vi "NsimuladotTemp.vi"(9 "Lmin":dbl, 10 "Lmax":dbl, 11 "N":i32) -> (3 "Array":dbl[](array[numeric]))   [LabVIEW 2020]
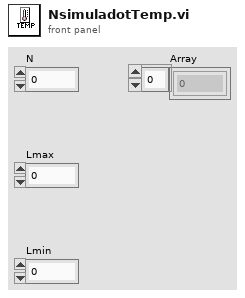
[diagram p1: front panel]
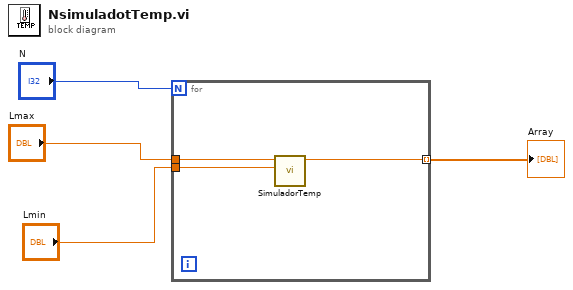
[diagram p0: block diagram]
diagram:
  n1 = for {
    N: "N" -> [_]
    tunnel: "Lmax" -> [w7]
    tunnel: "Lmin" -> [w6]
    tunnel: [w5] -> w4 mode=indexing
    n2 = call "SimuladorTemp.vi"("Lmin"=w6, "Lmax"=w7) -> ("Numeric"=w5:dbl)  [unwired: 9 in]
  }
  "Array" <- w4
